vi "DAQ VI(02-10-2020).vi"() -> ()   [LabVIEW 2020]
uses:
  <vilib>/DAQmx/read.llb/DAQmx Read (Analog 1D Wfm NChan NSamp).vi
  <vilib>/DAQmx/miscellaneous.llb/DAQmx Fill In Error Info.vi
panel:
  out "data":waveform(dbl)[](array[waveform])
  in  "number of samples per channel":i32=-1
  out "Waveform Graph":waveform(dbl)[](graph)
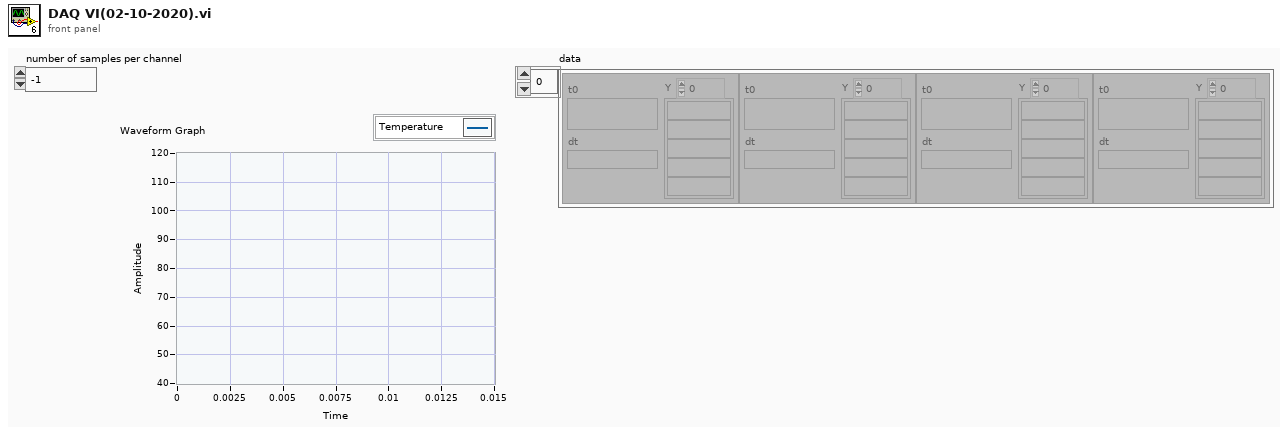
[diagram p1: front panel]
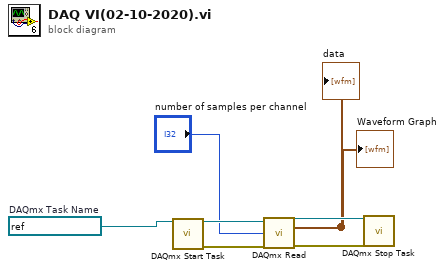
[diagram p0: block diagram]
diagram:
  w7 = refnum<k21> "NCNS Temp"  # DAQmx Task Name
  n1 = call <vilib>:"DAQmx Start Task.vi"("task/channels in"=w7) -> ("task out"=w6:refnum<k21>, "error out"=w4:errorcluster)  [unwired: 13 in]
  n2 = call-poly <vilib>:"DAQmx Read.vi"("task/channels in"=w6, "number of samples per channel"="number of samples per channel", "error in"=w4) -> ("task out"=w5:refnum<k21>, "data"=→"Waveform Graph" →"data":waveform(dbl)[], "error out"=w3:errorcluster)  [unwired: 10 in]
  n3 = call <vilib>:"DAQmx Stop Task.vi"("task/channels in"=w5, "error in"=w3) -> ()  [unwired: 12 in, 2 out]
